vi "TEST - Mangle VI Name.vi"(8 "error in (no error)":errorcluster) -> (0 "error out":errorcluster, 2 "pass":bool)   [LabVIEW 2009]
uses:
  source/library/UnMangle VI Name/UnMangle VI Name (String).vi
  source/library/Mangle VI Name/Mangle VI Name (String).vi
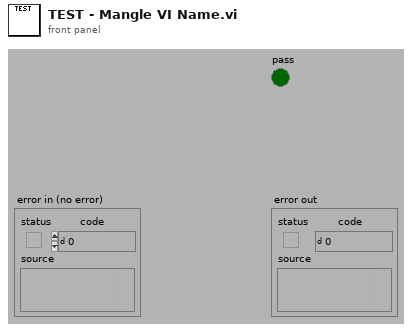
[diagram p1: front panel]
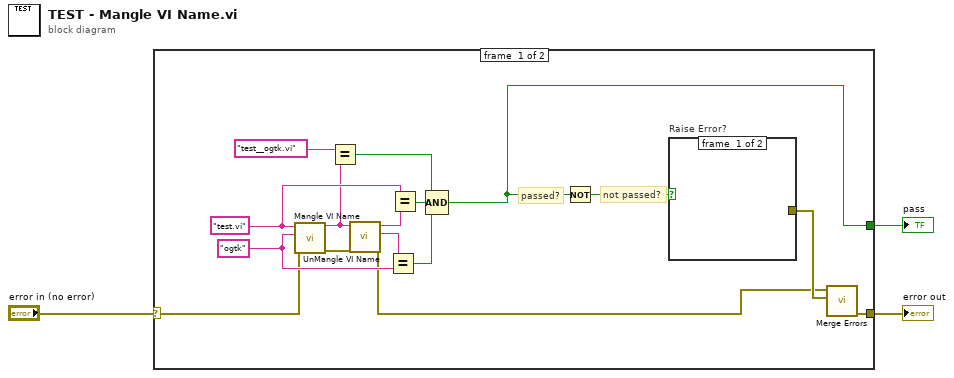
[diagram p0: block diagram]
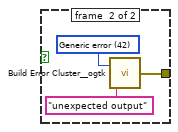
[diagram p2: hidden frame]
diagram:
  n1 = case shown="No Error" "error in (no error)" {
    selector: "error in (no error)" -> [w5 w23]
    tunnel: [w4 _] -> w3
    tunnel: [w19 w23] -> w1
    frame #0 {
      w12 = "ogtk" ("x")
      w14 = "test.vi" ("x")
      # "not passed?"
      # "passed?"
      n2 = call-poly "Mangle VI Name.vi"("error in (no error)"=w5, "Namespace (\"\": don't mangle)"=w12, "Name"=w14) -> ("error out"=w16:errorcluster, "Mangled Name"=w11:string)  [unwired: 7 in]
      n3 = Equal?(x="test__ogtk.vi", y=w11) -> (x = y?=w9:bool)
      n4 = call-poly "UnMangle VI Name.vi"("error in (no error)"=w16, "Mangled Name"=w11) -> ("error out"=w6:errorcluster, "Namespace"=w13:string, "UnMangled Name"=w15:string)  [unwired: 7 in]
      n5 = Equal?(x=w13, y=w12) -> (x = y?=w8:bool)
      n6 = Equal?(x=w14, y=w15) -> (x = y?=w7:bool)
      n7 = Compound Arithmetic op=AND(w9, w7, w8) -> (w4:bool)
      n8 = Not(x=w4) -> (.not. x?=w17:bool)
      n9 = case "Raise Error?" shown="True" w17 {
        tunnel: [_ w20] -> w18
        frame #0 {
        }
        frame #1 {
          w21 = 42 items=["No error", "Argument error", "Memory is full", "Out of zone", "End of file", "File already open", "Generic file I/O error", "File not found", "File permission error", "Disk is full", "Duplicate path", "Too many files open", "System feature not enabled", "Resource file not found", "Cannot add resource", "Resource not found", "Image not found", "Image memory error", "Pen does not exist", "Config type invalid", "Config token not found", "Config parse error", "Config memory error", "Bad external code format", "Bad external code offset", "External code not present", "Null window", "Destroy window error", "Null menu", "Print aborted", "Bad print record", "Print driver error", "Windows error during printing", "Memory error during printing", "Print dialog error", "Generic print error", "Invalid device refnum", "Device not found", "Device parameter error", "Device unit error", "Cannot open device", "Device call aborted", "Generic error", "Cancelled by user", "Object ID too low", "Object ID too high", "Object not in heap", "Unknown heap", "Unknown object (invalid DefProc)", "Unknown object (DefProc not in table)", "Message out of range", "Invalid (null) method", "Unknown message", "Manager call not supported", "Bad address", "Network operation in progress", "Network operation timed out", "Connection is busy", "Network attribute not supported", "Network error", "Address in use", "System out of memory", "Connection aborted", "Connection refused", "Not connected", "Already connected", "Connection closed", "Initialization error (interapplication manager)", "Bad occurrence", "Wait on unbound occurrence handler", "Occurrence queue overflow", "Datalog type conflict", "Unused", "Unrecognized type (interapplication manager)", "Memory corrupt", "Failed to make temporary DLL", "Old CIN version", "Drag socket not found", "Failed to load drop-object", "Failed to register OLE object", "Failed to release OLE object", "Format specifier type mismatch", "Unknown format specifier", "Too few format specifiers", "Too many format specifiers", "Scan failed", "Newer CIN version", "Error converting to variant", "Runtime menu error", "Password tampered", "Variant attribute not found", "Incompatible variant data type", "Event data is not available", "Event Store is not present", "Occurrence is not found", "Event Queue is not created", "Event info is not available", "Refnum passed is NULL", "Error retrieving Class GUID", "Error retrieving CoClass GUID", "Error retrieving TypeLib GUID.", "Bad built application magic bytes.", "Specific driver is different from the specific driver associated with the Logical Name.", "There is no session opened to the class driver.", "Max Error", "MAX - Error with config objects", "MAX - Error loading configuration", "MAX - Group not supported"]
          n10 = call <userlib>:"Build Error Cluster__ogtk.vi"("String to Prepend to source (\"\")"="unexpected output" ("String to Prepend to source (\"\")"), "code"=w21) -> ("error out"=w20:errorcluster)
        }
      }
      n11 = call <vilib>:"Merge Errors.vi"("error in 2 (no error)"=w18, "error in 1 (no error)"=w6) -> ("error out"=w19:errorcluster)  [unwired: 5 in]
    }
    frame #1 {
    }
  }
  "pass" <- w3
  "error out" <- w1
